vi "设定圆心与半径.vi"(8 "error in (no error)":errorcluster caption="错误输入（无错误）", 9 "半径":dbl=1.0, 10 "圆心":T1 caption="点", 11 "圆形 输入":refnum<class "圆形.lvclass"> caption="DNL_LabVIEW Object in") -> (0 "error out":errorcluster caption="错误输出", 3 "圆形 输出":refnum<class "圆形.lvclass"> caption="DNL_LabVIEW Object out")   [LabVIEW 2011, in "圆形.lvclass"]
uses:
  <vilib>/Utility/miscctls.llb/LVPointDoubleTypeDef.ctl
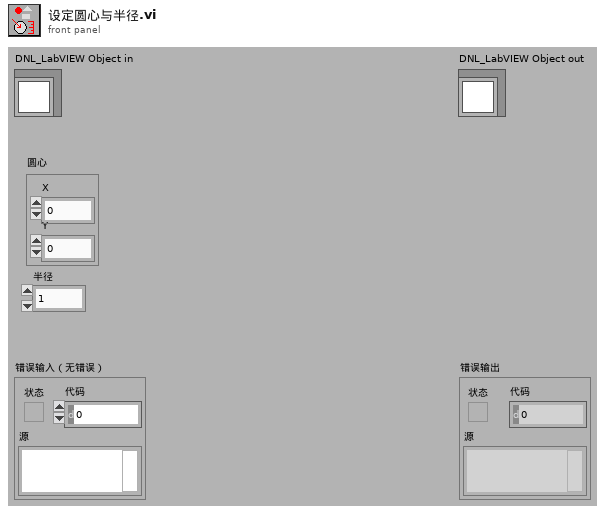
[diagram p1: front panel]
types:
  T1 = typedef "LVPointDoubleTypeDef.ctl" = cluster{"X":dbl, "Y":dbl}
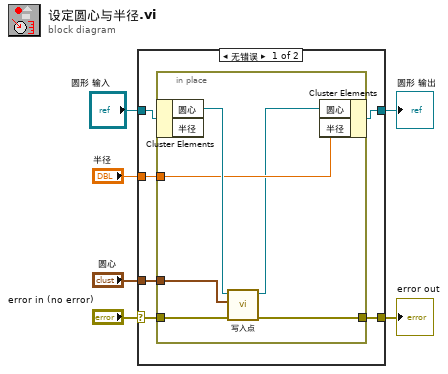
[diagram p0: block diagram]
diagram:
  n1 = case shown="无错误" "error in (no error)" {
    selector: "error in (no error)" -> [w10 w20]
    tunnel: [w7 w20] -> w5
    tunnel: [w9 w19] -> w3
    tunnel: "圆形 输入" -> [w12 w19]
    tunnel: "圆心" -> [w11 _]
    tunnel: "半径" -> [w8 _]
    frame No Error {
      n2 = in-place {
        in-place-border: w11 -> [w17]
        in-place-border: w10 -> [w16]
        in-place-border: w8 -> [w15]
        in-place-border: [w14] -> w7
        n3 = in-place-cluster #1(w12) -> ("圆心"=w18:refnum<class "点.lvclass">)  [unwired: 1 out]
        n4 = call "写入点.vi"("error in (no error)"=w16, "点"=w17, "点输入"=w18) -> ("error out"=w14:errorcluster, "点输出"=w13:refnum<class "点.lvclass">)  [unwired: 7 in]
        n5 = in-place-cluster #1("圆心"=w13, "半径"=w15) -> (w9:refnum<class "圆形.lvclass">)
      }
    }
    frame Error {
    }
  }
  "error out" <- w5
  "圆形 输出" <- w3
